vi "getRampParameters.vi"(8 "error in (no error)":errorcluster, 11 "RampEvent in":refnum<class "RampEvent.lvclass">) -> (0 "error out":errorcluster, 2 "RampParameters":T1, 3 "RampEvent out":refnum<class "RampEvent.lvclass">)   [LabVIEW 2009, in "Tools.lvlib" / "Scripting.lvlib" / "RampEvent.lvclass"]
uses:
  RampEvent.lvclass
  RampEvent.lvclass/RampEvent.ctl
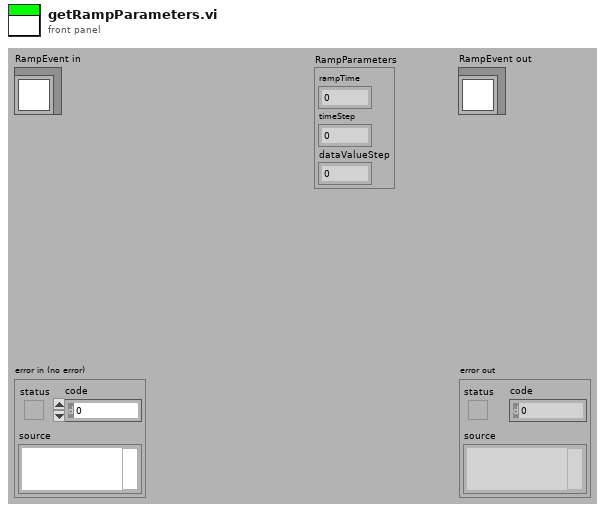
[diagram p1: front panel]
types:
  T1 = cluster{"rampTime":dbl, "timeStep":dbl, "dataValueStep":dbl}
  T2 = cluster{"rampTime":dbl, "timeStep":dbl, "valueStep":dbl}
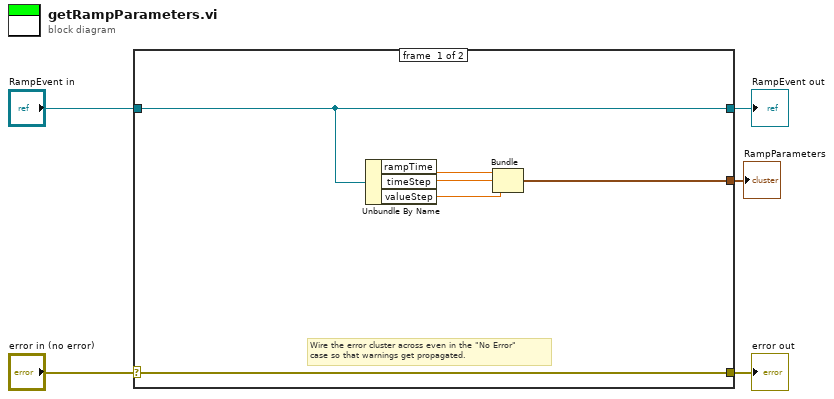
[diagram p0: block diagram]
diagram:
  n1 = case shown="No Error" "error in (no error)" {
    selector: "error in (no error)" -> [w11 w13]
    tunnel: [w11 w13] -> w4
    tunnel: [w7 w12] -> w2
    tunnel: "RampEvent in" -> [w7 w12]
    tunnel: [w6 _] -> w1
    frame #0 {
      # "Wire the error cluster across even in the \"No Error\"\ncase so that warnings get propagated."
      n2 = Unbundle By Name(w7) -> ("rampTime"=w10:dbl, "timeStep"=w9:dbl, "valueStep"=w8:dbl)
      n3 = Bundle("rampTime"=w10, "timeStep"=w9, "valueStep"=w8) -> (w6:T2)  [unwired: 1 in]
    }
    frame #1 {
    }
  }
  "error out" <- w4
  "RampEvent out" <- w2
  "RampParameters" <- w1
